vi "Waveform 2 Sub VI (FINAL).vi"(0 "error in (no error)":errorcluster, 3 "VISA Refnum in":refnum<visa-resource-name>) -> (1 "error out":errorcluster, 2 "Array":dbl[](array[numeric]))   [LabVIEW 2017]
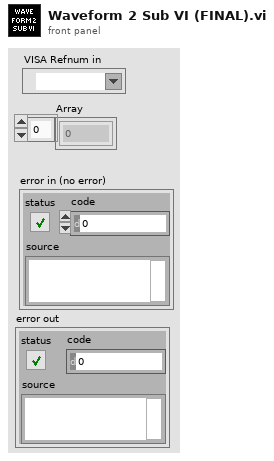
[diagram p1: front panel]
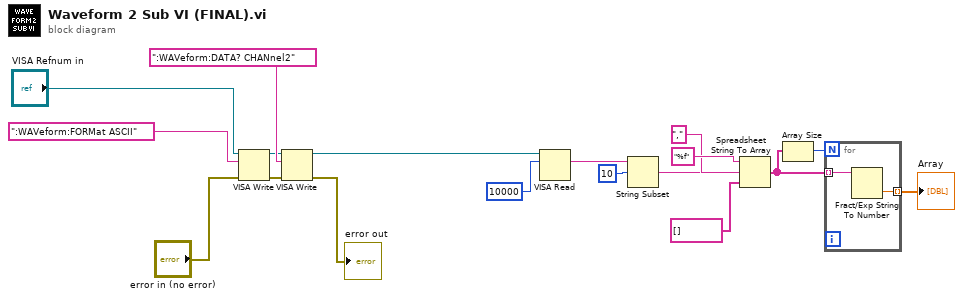
[diagram p0: block diagram]
diagram:
  n1 = VISA Write(VISA resource name="VISA Refnum in", write buffer=":WAVeform:FORMat ASCII", error in (no error)="error in (no error)") -> (VISA resource name out=w4:refnum<visa-resource-name>, error out=w3:errorcluster)  [unwired: 1 out]
  n2 = VISA Write(VISA resource name=w4, write buffer=":WAVeform:DATA? CHANnel2", error in (no error)=w3) -> (VISA resource name out=w8:refnum<visa-resource-name>, error out=→"error out":errorcluster)  [unwired: 1 out]
  n3 = VISA Read(VISA resource name=w8, byte count=u32 10000) -> (read buffer=w14:string)  [unwired: 1 in, 3 out]
  n4 = String Subset(string=w14, offset (0)=10) -> (substring=w12:string)  [unwired: 1 in]
  n5 = Spreadsheet String To Array(delimiter (Tab)="," ("spreadsheet string"), format string="%f", spreadsheet string=w12, array type (2D Dbl)=string[] []) -> (array=w10:string[])
  n6 = Array Size(array=w10) -> (size(s)=w11:i32)
  n7 = for {
    N: w11 -> [_]
    tunnel: w10 -> [w20] mode=indexing
    tunnel: [w19] -> w9 mode=indexing
    n8 = Fract/Exp String To Number(string=w20) -> (number=w19:dbl)  [unwired: 3 in, 1 out]
  }
  "Array" <- w9
